vi "CalStruct_IncrementNumCals.vi"(8 "error in":errorcluster) -> (0 "error out":errorcluster, 3 "Return Code":i32)   [LabVIEW 2015]
doc: "Description:\nThis function will increment the \"Number of Calibrations\" variable in the local EEPROM structure.\nDetail:\nint CalStruct_IncrementNumCals (\nvoid \n);\nParameters:\nNone\n\nReturn Values:\nThis function returns a 0 if the function completed successfully. A non-zero return code will indicate error. \nRemarks:\nCall this function when all calibrations have completed successfully, and before the data is written back to the DSP EEPROM."
uses:
  ScannerDiagDLL.dll
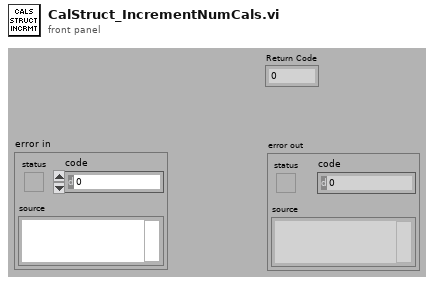
[diagram p1: front panel]
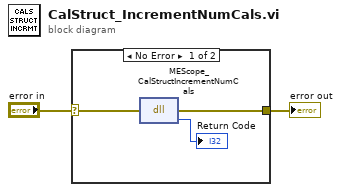
[diagram p0: block diagram]
diagram:
  n1 = case shown="No Error" "error in" {
    selector: "error in" -> [w5 w6]
    tunnel: [w4 w6] -> w1
    frame No Error {
      n2 = dll-call lib="C:/SNAPON/ModisEdge/TabletScope/Test Sequence/Code Modules/DLL/ScannerDiagDLL.dll" fn="MEScope_CalStructIncrementNumCals"(error in=w5) -> (error out=w4:errorcluster, "return type"=→"Return Code":i32)  [unwired: 2 in, 1 out]
    }
    frame Error {
    }
  }
  "error out" <- w1
